vi "IPI-VisionParam.vi"(8 "Vsion Param Set":string[][](array[string]), 11 "created path":path) -> ()   [LabVIEW 2015]
uses:
  <vilib>/Utility/file.llb/Write To Spreadsheet File (string).vi
panel:
  out "添加的路径":path
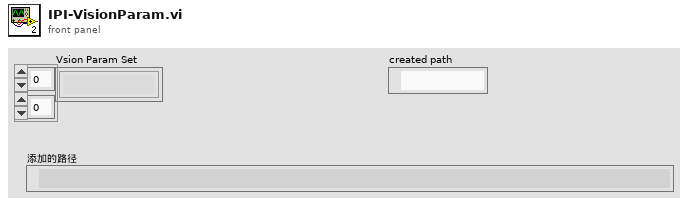
[diagram p1: front panel]
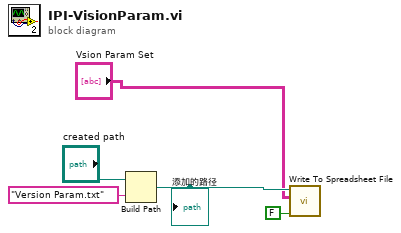
[diagram p0: block diagram]
diagram:
  n1 = Build Path(base path="created path", name or relative path="Version Param.txt" ("名称或相对路径")) -> (appended path=w3:path)
  "添加的路径" <- w3
  n2 = call-poly <vilib>:"Write To Spreadsheet File.vi"("append to file? (new file:F)"=FALSE, "2D data"="Vsion Param Set", "file path (dialog if empty)"=w3) -> ()  [unwired: 5 in, 1 out]
